vi "Send Normal Stop.vi"(8 "error in (no error)":errorcluster, 11 "Message Enqueuer":refnum<class "Message Enqueuer.lvclass">) -> (0 "error out":errorcluster)   [LabVIEW 2020, in "Actor Framework.lvlib" / "Stop Msg.lvclass"]
doc: "<p>(<strong>Filename</strong>: <span class=\"dnl\">Actor Framework.lvlib:Stop Msg.lvclass:Send Normal Stop.vi</span>)</p>\n\n<p>Sends a Stop message to an actor, triggering the actor to run its Stop Core method. This message has normal priority, meaning the actor will process this message after processing high- or normal-priority messages that are in the queue already.</p>"
uses:
  Stop Msg.lvclass
  Message Enqueuer/Message Enqueuer.lvclass
  C:/justACS/Actor Framework/Core/ActorFramework/Message/Message.lvclass
  Message Enqueuer/Message Enqueuer.lvclass/Message Enqueuer.ctl
  <vilib>/Utility/LVClass/Get LV Class Name.vi
  tracing/Trace Generation/Generate Trace for Message.vi
  Message Priority Queue/Priority Enqueue.vi
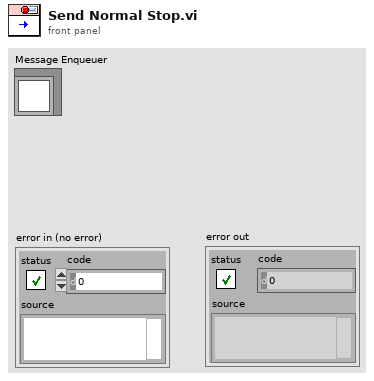
[diagram p1: front panel]
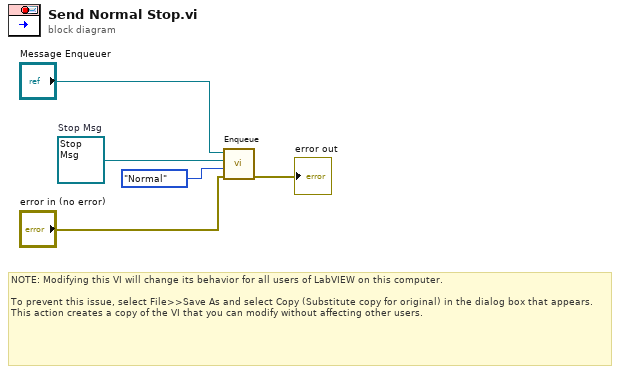
[diagram p0: block diagram]
diagram:
  w4 = refnum<class "Stop Msg.lvclass"> refnum  # Stop Msg
  # "NOTE: Modifying this VI will change its behavior for all users of LabVIEW on this computer.\n\nTo prevent this issue, select File>>Save As and select Copy (Substitute copy for original) in the dialog box that appears. This action creates a copy of the VI that you can modify without affecting other users."
  n1 = call "Enqueue.vi"("error in (no error)"="error in (no error)", "Message Priority (Normal)"=enum16{"Low", "Normal", "High"}."Normal" ("Queue Priority (Normal)"), "Message"=w4, "Message Enqueuer in"="Message Enqueuer") -> ("error out"=→"error out":errorcluster)  [unwired: 6 in, 1 out]
